vi "Get Pixel Size.vi"(8 "error in (no error)":errorcluster, 10 "ySize":sgl, 11 "xSize":sgl) -> (0 "error out":errorcluster, 1 "function return":u32, 2 "ySize out":sgl, 3 "xSize out":sgl)   [LabVIEW 2014, in "atmcd32d.lvlib"]
doc: "unsigned int WINAPI GetPixelSize(float * xSize, float * ySize);"
uses:
  atmcd32d.lvlib
  atmcd32d.dll
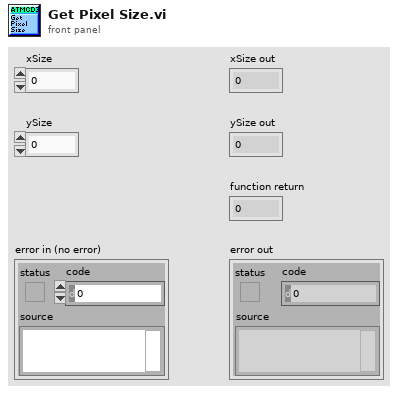
[diagram p1: front panel]
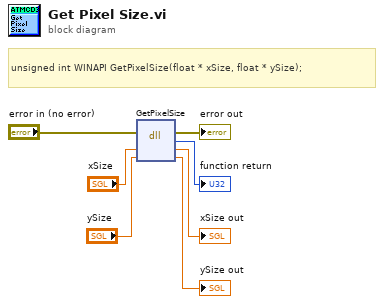
[diagram p0: block diagram]
diagram:
  # "unsigned int WINAPI GetPixelSize(float * xSize, float * ySize);"
  n1 = dll-call lib="C:/Users/Bakir/Documents/Lambda2-Testing/lib/Andorlib/atmcd32d.*" fn="GetPixelSize"(error in="error in (no error)", "xSize"="xSize", "ySize"="ySize") -> (error out=→"error out":errorcluster, →"function return":u32, "xSize"=→"xSize out":sgl, "ySize"=→"ySize out":sgl)  [unwired: 2 in, 1 out]
